vi "DAQ_pp3b_stateToMaster9Int.vi"(11 "State In":T1={"Curr  tr"=0, "Curr (ms)"=0, "Cum (ms)"=0, "Run loop diff"=0, "Tone countdown (ms)"=0, "Countdown (ms)"=0, "Curr State"=enum."0 NULL", "Prev State"=enum."0 NULL", "Rw"=FALSE, "Sw"=FALSE, "Tone\nGate"=FALSE, "Punish"=FALSE, "Current DAQ DO Int"=0, "Current Loaded Trial"={"Trial Type Number"=1, "Trial Type"=enum."GO", "Trial Weight"=100, "Shock (mA)"=0.3, "Duration (ms)"=0.25, "Sound Type"=enum."04 FM Sweep", "Stim P1"=4000.0, "Stim P2"=0.0, "Stim P3"=0.0, "Stim P4"=2000.0, "DAQ Amplitude (V)"=0.25}, "Total trials memo"=0, "State start cum memo (ms)"=0, "Last dur jump time memo (ms)"=0, "Last dur shock time memo (ms)"=0, "Tone repeat memo (ms)"=0, "Webcam on"=FALSE, "Webcam recording"=FALSE, "State update flag"=FALSE, "Last loaded shock voltage"=0.0, "Vid upd"=enum."0", "First time tone"=FALSE} {"Current DAQ DO Int" format="%016b"; "Current Loaded Trial"."DAQ Amplitude (V)" min=0.0 max=5.0 format="%_4g"; "Current Loaded Trial"."Shock (mA)" min=-1.0 max=5.0; "Current Loaded Trial"."Trial Weight" step=1; "Current Loaded Trial"."Duration (ms)" min=0.0 max=1.0; "Current Loaded Trial"."Trial Type Number" min=1 max=256 step=1}) -> (3 "Master-9 Output Array":bool[](array[boolean]))   [LabVIEW 2013]
uses:
  CTL_pp3c_LoopState.ctl
  pp3_CTL_BehavioralState.ctl
  pp3_CTL_Trial.ctl
  pp3_CTL_TrialType.ctl
  labolabo2/waveforms/WFTypes.ctl
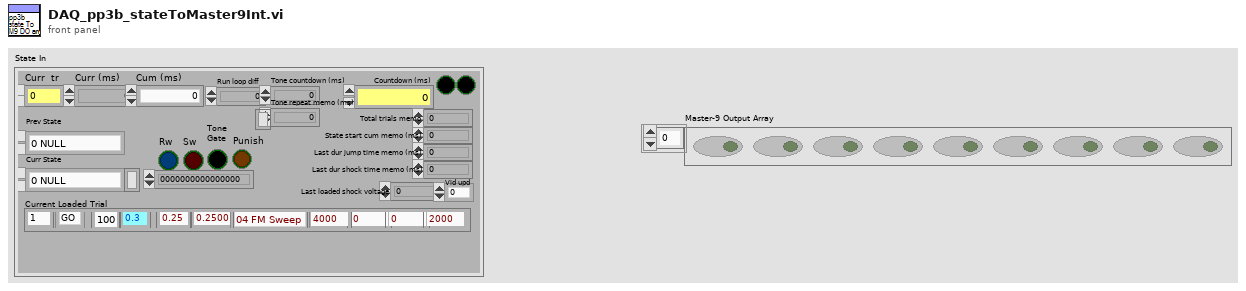
[diagram p1: front panel]
types:
  T1 = typedef "CTL_pp3c_LoopState.ctl" = cluster{"Curr  tr":u16, "Curr (ms)":u32, "Cum (ms)":u64, "Run loop diff":i64, "Tone countdown (ms)":i64, "Countdown (ms)":i64, "Curr State":T2, "Prev State":T2, "Rw":bool, "Sw":bool, "Tone\nGate":bool, "Punish":bool, "Current DAQ DO Int":u16, "Current Loaded Trial":T3, "Total trials memo":i64, "State start cum memo (ms)":i64, "Last dur jump time memo (ms)":i64, "Last dur shock time memo (ms)":i64, "Tone repeat memo (ms)":i64, "Webcam on":bool, "Webcam recording":bool, "State update flag":bool, "Last loaded shock voltage":dbl, "Vid upd":enum16{"0", "1", "2", "3", "4", "5", "6", "7", "8", "9"}, "First time tone":bool}
  T2 = typedef "pp3_CTL_BehavioralState.ctl" = enum8{"0 NULL", "1 Habituation", "2 (Load Trial)", "3 Stay Period", "4 Load Audio/Click Delay", "5 GO Trial", "6 GO Jumped", "7 GO Timeout", "8 NOGO Trial", "9 NOGO Jumped", "10 NOGO Timeout", "11 TEST Trial", "12 TEST Jumped", "13 TEST Timeout", "14 Intertrial Interval", "15 Done"}
  T3 = typedef "pp3_CTL_Trial.ctl" = cluster{"Trial Type Number":i16, "Trial Type":T4, "Trial Weight":u32, "Shock (mA)":dbl, "Duration (ms)":dbl, "Sound Type":T5, "Stim P1":dbl, "Stim P2":dbl, "Stim P3":dbl, "Stim P4":dbl, "DAQ Amplitude (V)":dbl}
  T4 = typedef "pp3_CTL_TrialType.ctl" = enum16{"OFF", "GO", "NOGO", "TEST"}
  T5 = typedef "WFTypes.ctl" = enum16{"00 NULL", "01 DC", "02 Noise", "03 Pure Tone", "04 FM Sweep"}
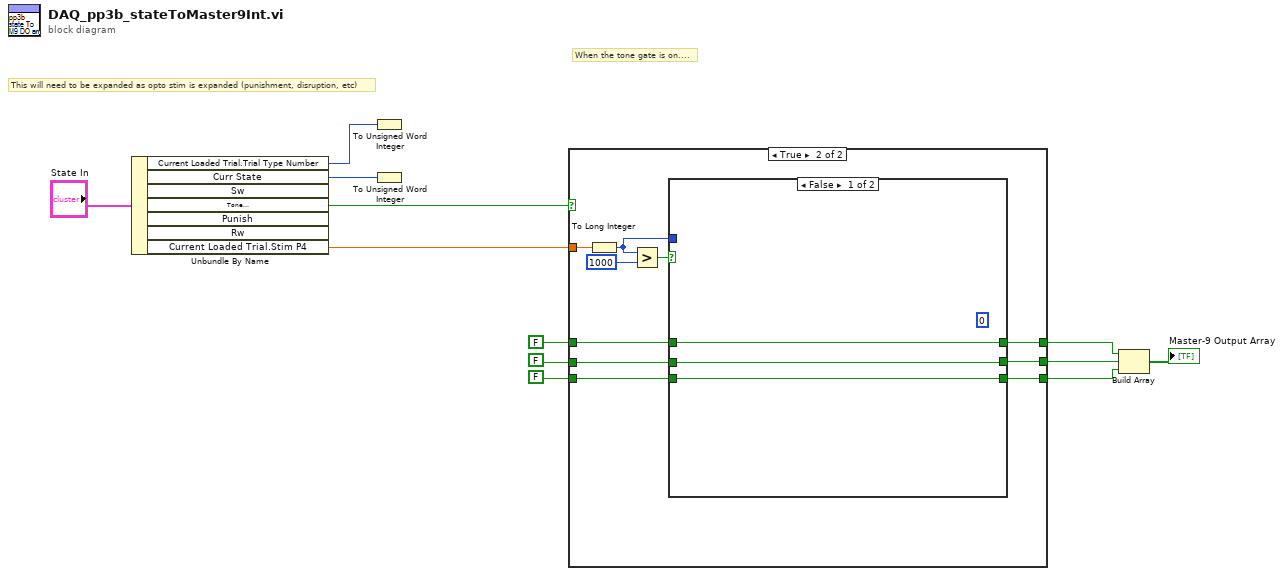
[diagram p0: block diagram]
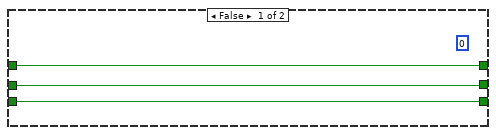
[diagram p2: hidden frame]
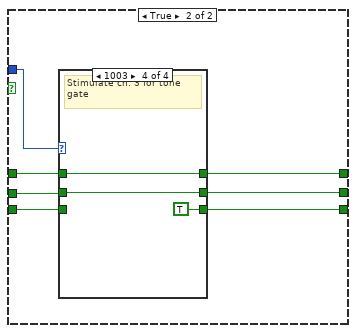
[diagram p3: hidden frame]
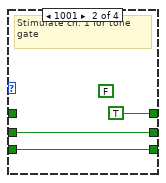
[diagram p5: hidden frame]
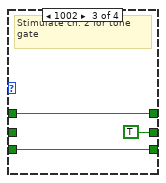
[diagram p6: hidden frame]
diagram:
  # "When the tone gate is on...."
  # "This will need to be expanded as opto stim is expanded (punishment, disruption, etc)"
  n1 = Unbundle By Name("State In") -> ("Current Loaded Trial.Trial Type Number"=w11:i16, "Curr State"=w10:T2, "Tone\nGate"=w9:bool, "Current Loaded Trial.Stim P4"=w8:dbl)  [unwired: 3 out]
  n2 = To Unsigned Word Integer(number=w11) -> ()  [unwired: 1 out]
  n3 = To Unsigned Word Integer(number=w10) -> ()  [unwired: 1 out]
  n4 = case shown="True" w9 {
    tunnel: w8 -> [_ w25]
    tunnel: [w15 w21] -> w6
    tunnel: [w14 w20] -> w5
    tunnel: [w13 w19] -> w4
    tunnel: FALSE -> [w15 w18]
    tunnel: FALSE -> [w14 w17]
    tunnel: FALSE -> [w13 w16]
    frame False {
      (unwired) u16 0 ("Master-9 Output Int")
    }
    frame True {
      n5 = To Long Integer(number=w25) -> (32bit integer=w22:i32)
      n6 = Greater?(x=w22, y=1000) -> (0:w23:bool)
      n7 = case shown="False" w23 {
        tunnel: w22 -> [_ w35]
        tunnel: [w28 w34] -> w21
        tunnel: [w27 w33] -> w20
        tunnel: [w26 w32] -> w19
        tunnel: w18 -> [w28 w31]
        tunnel: w17 -> [w27 w30]
        tunnel: w16 -> [w26 w29]
        frame False {
          (unwired) u16 0 ("Master-9 Output Int")
        }
        frame True {
          n8 = case shown="1003" w35 {
            tunnel: [w38 TRUE w44 w47] -> w34
            tunnel: [w37 w41 TRUE w46] -> w33
            tunnel: [w36 w40 w43 TRUE] -> w32
            tunnel: w31 -> [w38 _ w44 w47]
            tunnel: w30 -> [w37 w41 _ w46]
            tunnel: w29 -> [w36 w40 w43 _]
            frame 0, Default {
            }
            frame 1001 {
              (unwired) FALSE
              # "Stimulate ch. 1 for tone gate"
            }
            frame 1002 {
              # "Stimulate ch. 2 for tone gate"
            }
            frame 1003 {
              # "Stimulate ch. 3 for tone gate"
            }
          }
        }
      }
    }
  }
  n9 = Build Array(w6, w5, w4) -> (→"Master-9 Output Array":bool[])
